vi "SparkfunRazorImu.vi"() -> ()   [LabVIEW 2019]
uses:
  <vilib>/Analysis/Matrix/Datatypes/RealMatrix.ctl
  <vilib>/Analysis/baseanly.llb/Mean (DBL).vi
  <vilib>/Analysis/baseanly.llb/Real A x B.vi
  <vilib>/Instr/_visa.llb/VISA Configure Serial Port (Instr).vi
  MadgwickAhrsWfmArray.vi
  <vilib>/Analysis/Matrix/Numeric/Conversions/Array To Matrix - RA2.vi
  <vilib>/Analysis/Matrix/Numeric/Conversions/Array To Matrix - RA.vi
  <vilib>/Analysis/Matrix/NI_Matrix.lvlib
  <vilib>/Analysis/NI_AALBase.lvlib
  MadgwickOrientationFilter.lvlib
  <vilib>/picture/3D Picture Control/NI_3D Picture Control.lvlib
panel:
  out "Roll":dbl
  out "Pitch":dbl
  out "Yaw":dbl
  out "Scene Display":refnum<vi>(3d-picture)
  out "A x B":T1
  out "Waveform Chart":waveform(dbl)[](graph)
  out "error out":errorcluster
  in  "stop":bool
  in  "error in":errorcluster
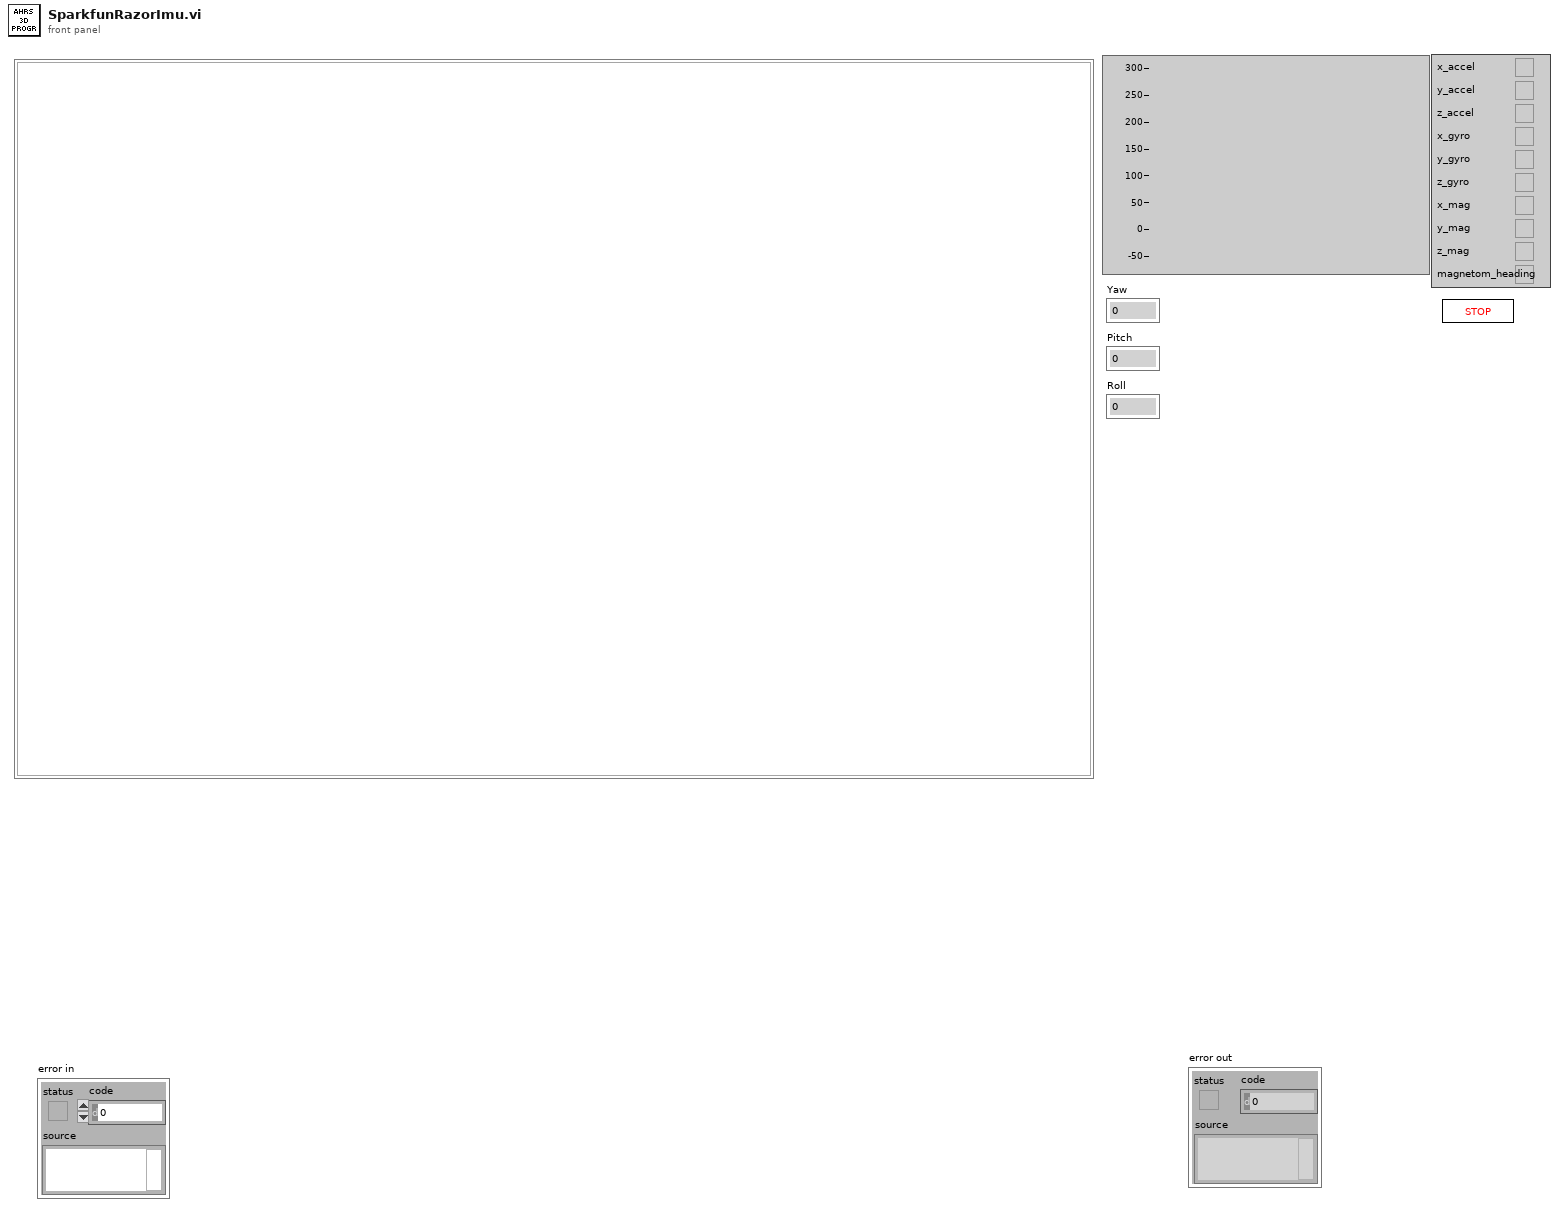
[diagram p1: front panel]
types:
  T1 = typedef "NI_Matrix.lvlib/RealMatrix.ctl" = dbl[][]
  T2 = cluster{"Red":sgl, "Green":sgl, "Blue":sgl, "Alpha":sgl}
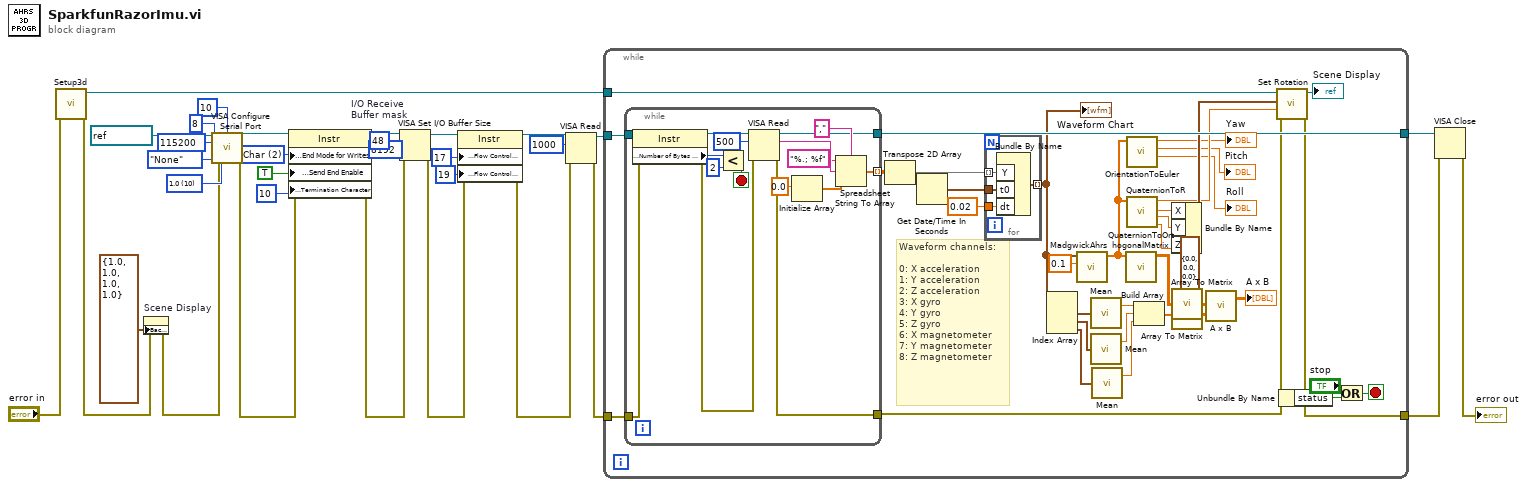
[diagram p0: block diagram]
diagram:
  w19 = u16 48  # I/O Receive Buffer mask
  w5 = u16 2 items=["None", "LastBit", "TermChar", "Break"] ("Serial Settings:Serial End Mode for Writes")
  w27 = u16 10 items=["1.0"=10, "1.5"=15, "2.0"=20] ("stop bits (10: 1 bit)")
  n1 = call "Setup3d.vi"("error in"="error in") -> ("error out"=w3:errorcluster, "Scene Object"=w1:refnum<vi>)  [unwired: 9 in]
  n2 = property on="Scene Display" class="SceneGraphDisp (strict)"(error in=w3, "Background Color"=T2 {"Red"=1.0, "Green"=1.0, "Blue"=1.0, "Alpha"=1.0}) -> (error out=w2:errorcluster)  [unwired: 1 in, 1 out]
  n3 = call-poly "VISA Configure Serial Port"("VISA resource name"=refnum<visa-resource-name> "COM1", "termination char\n(0xA = '\\n' = LF)"=u8 10 ("termination char\n(0xA = '\\n' = LF)"), "baud rate (9600)"=u32 115200, "data bits (8)"=u16 8, "parity (0:none)"=enum16{"None", "Odd", "Even", "Mark", "Space"}."None", "error in (no error)"=w2, "stop bits (10: 1 bit)"=w27) -> ("VISA resource name out"=w11:refnum<visa-resource-name>, "error out"=w10:errorcluster)  [unwired: 7 in]
  n4 = property class="Instr"(reference=w11, error in=w10, "Serial Settings:End Mode for Writes"=w5, "Message Based Settings:Send End Enable"=TRUE, "Message Based Settings:Termination Character"=u8 10 ("termination char\n(0xA = '\\n' = LF)")) -> (reference out=w17:refnum<visa-resource-name>, error out=w9:errorcluster)
  n5 = VISA Set I/O Buffer Size(VISA resource name=w17, mask (16)=w19, size (4096)=u32 8192 ("Input\nbuffer size"), error in (no error)=w9) -> (VISA resource name out=w14:refnum<visa-resource-name>, error out=w8:errorcluster)
  n6 = property class="Instr"(reference=w14, error in=w8, "Serial Settings:Flow Control XON Character"=u8 17 ("XON Character"), "Serial Settings:Flow Control XOFF Character"=u8 19 ("XOFF Character")) -> (reference out=w13:refnum<visa-resource-name>, error out=w7:errorcluster)
  n7 = VISA Read(VISA resource name=w13, byte count=u32 1000, error in (no error)=w7) -> (VISA resource name out=w4:refnum<visa-resource-name>, error out=w6:errorcluster)  [unwired: 2 out]
  n8 = while {
    tunnel: [w41] -> w23
    tunnel: w6 -> [w46]
    tunnel: w1 -> [w45]
    tunnel: w4 -> [w51]
    tunnel: [w47] -> w24
    stop <- w53 stop-if-true
    # "Waveform channels:\n\n0: X acceleration\n1: Y acceleration\n2: Z acceleration\n3: X gyro\n4: Y gyro\n5: Z gyro\n6: X magnetometer\n7: Y magnetometer\n8: Z magnetometer"
    n9 = while {
      tunnel: [w77] -> w49 mode=indexing
      tunnel: w51 -> [w83]
      tunnel: [w76] -> w42
      tunnel: [w75] -> w47
      tunnel: w46 -> [w74]
      stop <- w82 stop-if-true
      n10 = property class="Instr"(reference=w83, error in=w74) -> (reference out=w88:refnum<visa-resource-name>, error out=w87:errorcluster, "Serial Settings:Number of Bytes at Serial Port"=w86:u32)
      n11 = Less?(x=w86, y=u32 2) -> (x < y?=w82:bool)
      n12 = VISA Read(VISA resource name=w88, byte count=u32 500, error in (no error)=w87) -> (VISA resource name out=w75:refnum<visa-resource-name>, read buffer=w81:string, error out=w76:errorcluster)  [unwired: 1 out]
      n13 = Initialize Array(0.0) -> (w79:dbl[])  [unwired: 1 in]
      n14 = Spreadsheet String To Array(delimiter (Tab)=",", format string="%.; %f", spreadsheet string=w81, array type (2D Dbl)=w79) -> (array=w77:dbl[])
    }
    n15 = Transpose 2D Array(2D array=w49) -> (transposed array=w50:dbl[][])
    n16 = Get Date/Time In Seconds() -> (seconds since 1Jan1904=w48:timestamp)
    n17 = for {
      tunnel: w50 -> [w71] mode=indexing
      tunnel: w48 -> [w73]
      tunnel: 0.02 -> [w72]
      tunnel: [w70] -> w38 mode=indexing
      n18 = Bundle By Name("Y"=w71, "t0"=w73, "dt"=w72) -> (w70:waveform(dbl))  [unwired: 1 in]
    }
    "Waveform Chart" <- w38
    n19 = Index Array(array=w38) -> (element #1=w61:waveform(dbl), element #2=w60:waveform(dbl), element #3=w59:waveform(dbl))  [unwired: 3 in]
    n20 = call-poly "MadgwickAhrs.vi"("Beta"=0.1, "Waveforms"=w38) -> ("Quaternion"=w37:dbl[])  [unwired: 9 in]
    n21 = call-poly <vilib>:"Mean.vi"("X"=w61) -> ("mean"=w62:dbl)  [unwired: 1 out]
    n22 = call-poly <vilib>:"Mean.vi"("X"=w60) -> ("mean"=w63:dbl)  [unwired: 1 out]
    n23 = call-poly <vilib>:"Mean.vi"("X"=w59) -> ("mean"=w64:dbl)  [unwired: 1 out]
    n24 = call "QuaternionToOrthogonalMatrix.vi"("Quaternion"=w37) -> ("OrthogonalMatrix"=w54:dbl[][])  [unwired: 10 in]
    n25 = call "OrientationToEuler.vi"("Quaternion"=w37) -> ("Roll"=→"Roll":dbl, "Pitch"=→"Pitch":dbl, "Yaw"=→"Yaw":dbl)  [unwired: 8 in]
    n26 = call "QuaternionToR.vi"("Quaternion"=w37) -> ("Rz"=w55:dbl, "Ry"=w56:dbl, "Rx"=w57:dbl, "Theta"=w43:dbl)  [unwired: 7 in]
    n27 = Build Array(w62, w63, w64) -> (w65:dbl[])
    n28 = Bundle By Name(cluster=cluster{"X":sgl, "Y":sgl, "Z":sgl} {"X"=0.0, "Y"=0.0, "Z"=0.0} ("Axis"), "X"=w57, "Y"=w56, "Z"=w55) -> (w44:cluster{"X":sgl, "Y":sgl, "Z":sgl})
    n29 = call-poly <vilib>:"Array To Matrix.vi"("Real 2D Array"=w54) -> ("Real Matrix"=w67:T1)
    n30 = call-poly <vilib>:"Array To Matrix.vi"("Real 1D Array"=w65) -> ("Real Matrix (Column Vector)"=w68:T1)
    n31 = call-poly <vilib>:"A x B.vi"("B"=w68, "A"=w67) -> ("A x B"=→"A x B":T1)  [unwired: 1 out]
    n32 = call <vilib>:"Set Rotation.vi"("error in (no error)"=w42, "Angle"=w43, "Axis"=w44, "Scene Object"=w45) -> ("error out"=w41:errorcluster, "Rotated Scene Object"=→"Scene Display":refnum<vi>)  [unwired: 6 in]
    n33 = Unbundle By Name(w41) -> ("status"=w33:bool)
    n34 = Or(x="stop", y=w33) -> (x .or. y?=w53:bool)
  }
  n35 = VISA Close(VISA resource name=w24, error in (no error)=w23) -> (error out=→"error out":errorcluster)
